vi "BinDiff.vi"() -> ()   [LabVIEW 2012]
panel:
  out "Numeric":i32
  out "Waveform Chart":u8(graph)
  out "x = y?":bool
  out "data 2":string
  out "data":string
  in  "Path2":path
  in  "Path1":path
  # "751"
  # "x3"
  # "2360068"
  # "2360047"
  # "x3"
  # "4719366"
  # "9439573"
  # "4720162"
  # "9526003"
  # "x2"
  # "x4"
  # "6293023"
  # "6293820"
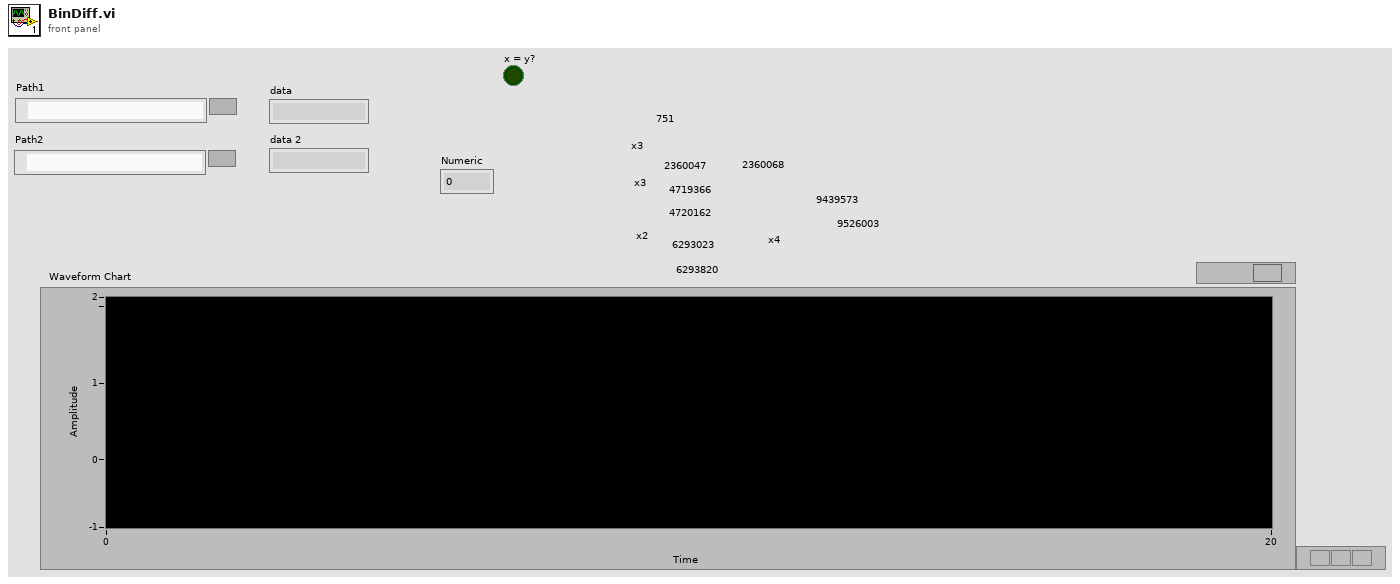
[diagram p1: front panel]
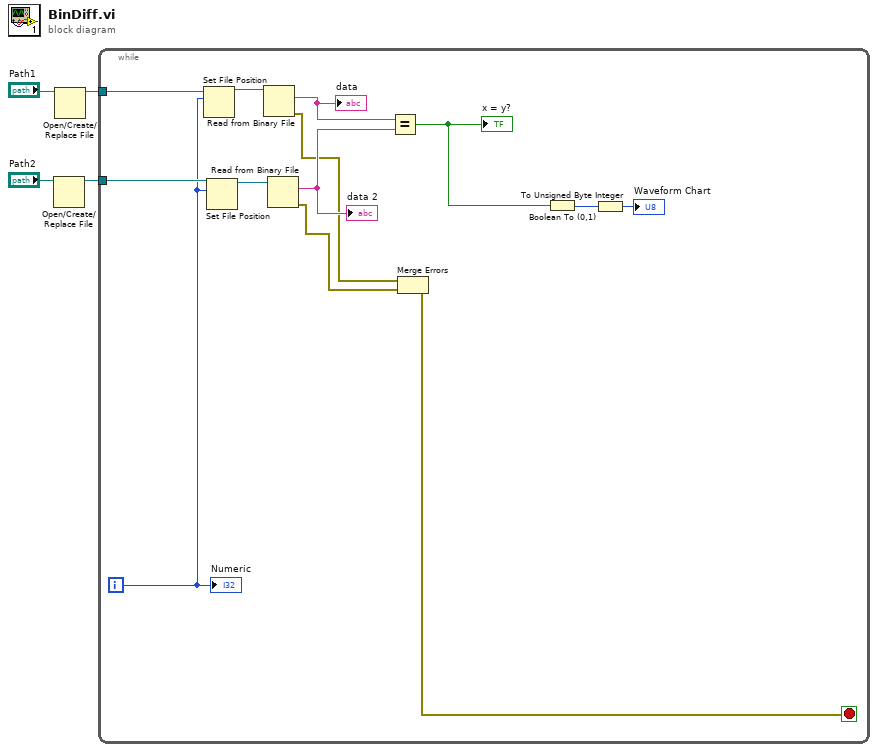
[diagram p0: block diagram]
diagram:
  n1 = Open/Create/Replace File(file path (use dialog)="Path2") -> (refnum out=w1:refnum<file>)  [unwired: 5 in, 2 out]
  n2 = Open/Create/Replace File(file path (use dialog)="Path1") -> (refnum out=w3:refnum<file>)  [unwired: 5 in, 2 out]
  n3 = while {
    tunnel: w1 -> [w13]
    tunnel: w3 -> [w14]
    i -> [w11]
    stop <- w8 stop-if-true
    n4 = Set File Position(offset (in bytes) (0)=w11, refnum=w14) -> (refnum out=w15:refnum<file>)  [unwired: 2 in, 1 out]
    n5 = Set File Position(offset (in bytes) (0)=w11, refnum=w13) -> (refnum out=w12:refnum<file>)  [unwired: 2 in, 1 out]
    n6 = Read from Binary File(11:w15) -> (0:w10:errorcluster, 2:w17:string)  [unwired: 5 in, 2 out]
    "data" <- w17
    n7 = Read from Binary File(11:w12) -> (0:w9:errorcluster, 2:w16:string)  [unwired: 5 in, 2 out]
    "data 2" <- w16
    n8 = Equal?(x=w17, y=w16) -> (x = y?=w5:bool)
    "x = y?" <- w5
    n9 = Merge Errors(w10, w9) -> (w8:errorcluster)
    n10 = Boolean To (0,1)(Boolean=w5) -> (0, 1=w7:i16)
    n11 = To Unsigned Byte Integer(number=w7) -> (unsigned 8bit integer=→"Waveform Chart":u8)
    "Numeric" <- w11
  }
